vi "Read Address.vi"(8 "error in":errorcluster, 11 "address ref in":refnum<k20>) -> (0 "error out":errorcluster, 2 "terminal":T1, 3 "address ref out":refnum<k20>)   [LabVIEW 2020, in "MIL-STD 1553 Import.lvlib"]
uses:
  MIL-STD 1553 Import.lvlib
  Shared/Terminal Endpoint.ctl
  Shared/Address.ctl
  997d6892-f520-484c-a71d-f8493dde3f6b.vi
  c4881378-0696-4b0e-820e-c01546609bba.vi
  285a92bc-9c63-43b3-b544-62fba9bc5a66.vi
  5052c8a8-a5e7-4770-b2a7-42c35e434072.vi
  997d6892-f520-484c-a71d-f8493dde3f6b.vi/b1e6fcf8-dac1-42d2-b1fe-151afe06dbd4.vi
  c4881378-0696-4b0e-820e-c01546609bba.vi/749400e4-5f60-4dbe-83d9-453db9d95f9d.vi
  c4881378-0696-4b0e-820e-c01546609bba.vi/472f3993-b042-455f-80f2-2140c22c21b8.vi
  c4881378-0696-4b0e-820e-c01546609bba.vi/3e45ab0b-a443-4555-805a-cc6dd0adbb20.vi
  285a92bc-9c63-43b3-b544-62fba9bc5a66.vi/b1e6fcf8-dac1-42d2-b1fe-151afe06dbd4.vi
  5052c8a8-a5e7-4770-b2a7-42c35e434072.vi/749400e4-5f60-4dbe-83d9-453db9d95f9d.vi
  5052c8a8-a5e7-4770-b2a7-42c35e434072.vi/472f3993-b042-455f-80f2-2140c22c21b8.vi
  5052c8a8-a5e7-4770-b2a7-42c35e434072.vi/3e45ab0b-a443-4555-805a-cc6dd0adbb20.vi
  997d6892-f520-484c-a71d-f8493dde3f6b.vi/b1e6fcf8-dac1-42d2-b1fe-151afe06dbd4.vi/49c1b1ee-2d2a-4a85-8ca5-42123c34e85a.vi
  c4881378-0696-4b0e-820e-c01546609bba.vi/749400e4-5f60-4dbe-83d9-453db9d95f9d.vi/49c1b1ee-2d2a-4a85-8ca5-42123c34e85a.vi
  c4881378-0696-4b0e-820e-c01546609bba.vi/472f3993-b042-455f-80f2-2140c22c21b8.vi/49c1b1ee-2d2a-4a85-8ca5-42123c34e85a.vi
  c4881378-0696-4b0e-820e-c01546609bba.vi/3e45ab0b-a443-4555-805a-cc6dd0adbb20.vi/49c1b1ee-2d2a-4a85-8ca5-42123c34e85a.vi
  285a92bc-9c63-43b3-b544-62fba9bc5a66.vi/b1e6fcf8-dac1-42d2-b1fe-151afe06dbd4.vi/49c1b1ee-2d2a-4a85-8ca5-42123c34e85a.vi
  5052c8a8-a5e7-4770-b2a7-42c35e434072.vi/749400e4-5f60-4dbe-83d9-453db9d95f9d.vi/49c1b1ee-2d2a-4a85-8ca5-42123c34e85a.vi
  5052c8a8-a5e7-4770-b2a7-42c35e434072.vi/472f3993-b042-455f-80f2-2140c22c21b8.vi/49c1b1ee-2d2a-4a85-8ca5-42123c34e85a.vi
  5052c8a8-a5e7-4770-b2a7-42c35e434072.vi/3e45ab0b-a443-4555-805a-cc6dd0adbb20.vi/49c1b1ee-2d2a-4a85-8ca5-42123c34e85a.vi
  Constants.vi
  Get Element References by Tag Name.vi
  <vilib>/xml/Get Node Text Content.vi
  <vilib>/Utility/error.llb/Error Cluster From Error Code.vi
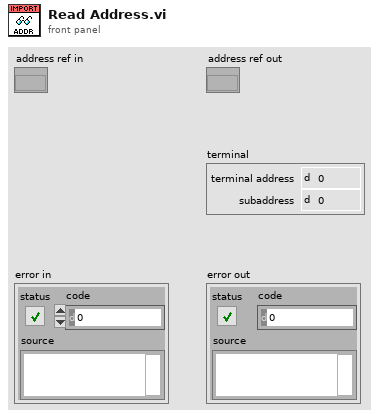
[diagram p1: front panel]
types:
  T1 = typedef "Terminal Endpoint.ctl" = cluster{"terminal address":T2, "subaddress":T2}
  T2 = typedef "Address.ctl" = u16
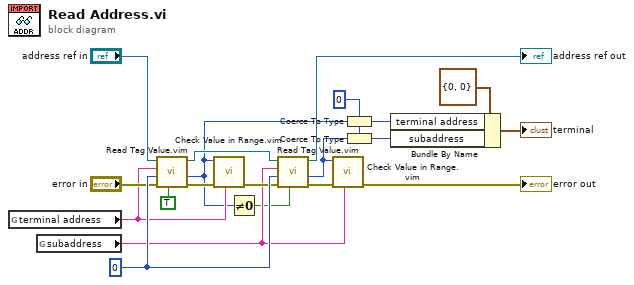
[diagram p0: block diagram]
diagram:
  w20 = u16 0 ("error code (0)")
  w17 = T2 0 ("subaddress")
  n1 = global read "Constants.vi" "terminal address"() -> (w4:string)
  n2 = global read "Constants.vi" "subaddress"() -> (w5:string)
  n3 = call "Read Tag Value.vim"("required (F)"=TRUE, "error in"="error in", "default"=w20, "tag name"=w4, "node in"="address ref in") -> ("error out"=w10:errorcluster, "value"=w2:u16, "node out"=w13:refnum<k20>)  [unwired: 4 in]
  n4 = call "Check Value in Range.vim"("element name"=w4, "error in"=w10, "value"=w2) -> ("error out"=w9:errorcluster)  [unwired: 8 in]
  n5 = Not Equal To 0?(x=w2) -> (x != 0?=w1:bool)
  n6 = call "Read Tag Value.vim"("required (F)"=w1, "error in"=w9, "default"=w20, "tag name"=w5, "node in"=w13) -> ("error out"=w8:errorcluster, "value"=w3:u16, "node out"=→"address ref out":refnum<k20>)  [unwired: 4 in]
  n7 = call "Check Value in Range.vim"("element name"=w5, "error in"=w8, "value"=w3) -> ("error out"=→"error out":errorcluster)  [unwired: 8 in]
  n8 = Coerce To Type(0:w2, 1:w17) -> (2:w15:T2)
  n9 = Coerce To Type(0:w3, 1:w17) -> (2:w16:T2)
  n10 = Bundle By Name(cluster=T1 {"terminal address"=0, "subaddress"=0} ("endpoint Rx"), "terminal address"=w15, "subaddress"=w16) -> (→"terminal":T1)
